vi "_FPGA Turbo Control.vi"(6 "error in (no error)":errorcluster, 8 "Command":T1=enum."Read Actual Rotation Speed in Hz") -> (0 "error out":errorcluster, 1 "Speed":i32, 2 "Reply":string, 4 "Error Code":string, 5 "Time":i32)   [LabVIEW 2012]
uses:
  Type/_Pump Parameter.ctl
  Type/_RT Serial Command.ctl
  _RT Global.vi
  <vilib>/Utility/error.llb/Error Cluster From Error Code.vi
  <vilib>/rvi/errors/niLvFpgaAdjustHostInterfaceError.vi
  <vilib>/rvi/interface/nirviReadWriteControl/nirviReadWriteControl.xnode
  FPGA Bitfiles/FPGA9602.lvbitx
  NiFpgaLv.dll
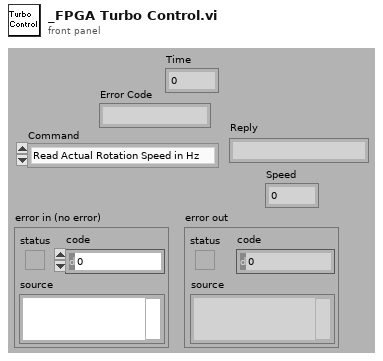
[diagram p1: front panel]
types:
  T1 = typedef "_Pump Parameter.ctl" = enum16{"Turn Pump Motor On", "Turn Pump Motor Off", "Read Pump Oil Deficiency", "Read Rotation Switch Point Attained", "Read Ele. Drive Over Temperature", "Read Pump Over Temperature", "Read Set Rotation Speed Attained", "Read Turbopump Accelerates", "Read Actual Rotation Speed in Hz", "Read Motor Current in A", "Read Operating Hours in h", "Read Motor Voltage in V", "Read Motor Power in W", "Set Rotation Speed Switchpoint in %", "Clear Error", "Read Error Code", "Read Bearing Temperature", "Read Hardware Version", "Read Firmware Version", "Read Operating Hours (Drive)", "Read Rotational Speed (rpm)", "Read Power Stage Temperature", "Read Electronics Temperature", "Read Upper Pump Temperature", "Read Motor Temperature", "Read Error Code History, 1", "Read Error Code History, 2", "Read Error Code History, 3", "Read Error Code History, 4", "Read Error Code History, 5", "Read Error Code History, 6", "Read Error Code History, 7", "Read Error Code History, 8", "Read Error Code History, 9", "Read Error Code History, 10"}
  T2 = typedef "_RT Serial Command.ctl" = cluster{"Port Type":u16, "baud rate (9600)":u32, "data bits (8)":u16, "stop bits (1)":u16, "parity (0:none)":u16, "DoRead":bool, "Command":string}
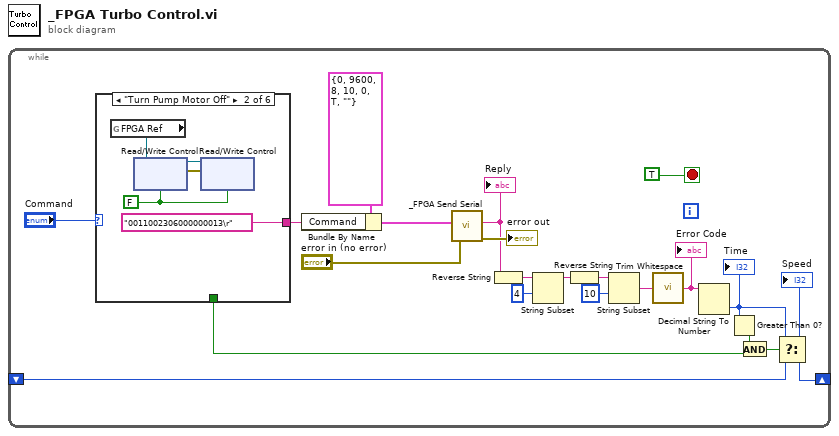
[diagram p0: block diagram]
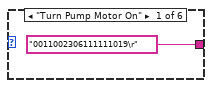
[diagram p2: hidden frame]
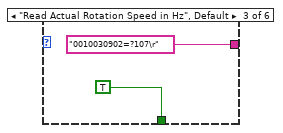
[diagram p3: hidden frame]
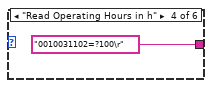
[diagram p4: hidden frame]
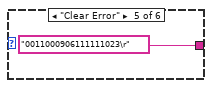
[diagram p5: hidden frame]
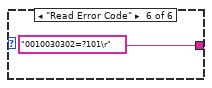
[diagram p6: hidden frame]
diagram:
  n1 = while {
    shift-right: [w2] -> _
    shift-left: _ -> [w3]
    stop <- TRUE stop-if-true
    n2 = case shown="\"Turn Pump Motor Off\"" "Command" {
      tunnel: ["0011002306111111019\r" ("Command") "0011002306000000013\r" ("Command") "0010030902=?107\r" ("Command") "0010031102=?100\r" ("Command") "0011000906111111023\r" ("Command") "0010030302=?101\r" ("Command")] -> w19
      tunnel: [_ _ TRUE _ _ _] -> w5
      frame "Turn Pump Motor On" {
      }
      frame "Turn Pump Motor Off" {
        w26 = FALSE
        n3 = global read "_RT Global.vi" "FPGA Ref"() -> (w23:refnum<k20>)
        n4 = xnode "Read/Write Control"("FPGA VI Reference In"=w23, "FilaB"=w26) -> ("FPGA VI Reference Out"=w24:refnum<k20>, "error out"=w25:errorcluster)  [unwired: 1 in]
        n5 = xnode "Read/Write Control"("FPGA VI Reference In"=w24, "error in"=w25, "FilaC"=w26) -> ()  [unwired: 2 out]
      }
      frame "Read Actual Rotation Speed in Hz", Default {
      }
      frame "Read Operating Hours in h" {
      }
      frame "Clear Error" {
      }
      frame "Read Error Code" {
      }
    }
    n6 = Bundle By Name(cluster=T2 {"Port Type"=0, "baud rate (9600)"=9600, "data bits (8)"=8, "stop bits (1)"=10, "parity (0:none)"=0, "DoRead"=TRUE, "Command"=""}, "Command"=w19) -> (w18:T2)
    n7 = call "_FPGA Send Serial.vi"("error in"="error in (no error)", "Serial Command"=w18) -> ("error out"=→"error out":errorcluster, "Reply"=w10:string)  [unwired: 2 in, 2 out]
    "Reply" <- w10
    n8 = Reverse String(1:w10) -> (0:w15:string)
    n9 = String Subset(string=w15, offset (0)=4) -> (substring=w11:string)  [unwired: 1 out]
    n10 = Reverse String(1:w11) -> (0:w12:string)
    n11 = String Subset(string=w12, offset (0)=10) -> (substring=w9:string)  [unwired: 1 out]
    n12 = call <vilib>:"Trim Whitespace.vi"("string"=w9) -> ("trimmed string"=w8:string)  [unwired: 1 in]
    "Error Code" <- w8
    n13 = Decimal String To Number(string=w8) -> (number=w1:i32)  [unwired: 3 out]
    "Time" <- w1
    n14 = Greater Than 0?(x=w1) -> (x > 0?=w6:bool)
    n15 = And(x=w6, y=w5) -> (x .and. y?=w4:bool)
    n16 = Select(t=w1, s=w4, f=w3) -> (s? t:f=w2:i32)
    "Speed" <- w2
  }
